vi "DDC Stage 02 - Single channel.vi"(0 "input cluster":T1={"acq.reset"=FALSE, "ddc.out.rate"=[0.0, 0.0, 0.0, 0.0, 0.0, 0.0, 0.0, 0.0, 0.0, 0.0, 0.0, 0.0, 0.0, 0.0, 0.0, 0.0], "ddc.delay"=[0.0, 0.0, 0.0, 0.0, 0.0, 0.0, 0.0, 0.0, 0.0, 0.0, 0.0, 0.0, 0.0, 0.0, 0.0, 0.0], "Channel#"=0} {"ddc.out.rate" format="%.48g"; "ddc.delay" format="%.16g"}, 7 "FIFO In":refnum<k21>="FIFO-000", 11 "Ch#":u8) -> (3 "dsp.overflow":bool, 4 "U32 out":u32, 10 "output valid":bool, 14 "dbg,output1":T2)   [LabVIEW 2015, in "DDC_7976R_v1.lvlib"]
uses:
  DDC_7976R_v1.lvlib
  Typedef - internal -03.ctl
  Typedef - internal -04.ctl
  <instrlib>/_niInstr/DSP/v1/FPGA/Public/Sub VIs/HB Decimator/Halfband Decimator - IQ - 16 spc - 2x oc.vi
  <instrlib>/_niInstr/DSP/v1/FPGA/Public/Sub VIs/HB Decimator/Halfband Decimator - IQ - 8 spc - 2x oc.vi
  <instrlib>/_niInstr/DSP/v1/FPGA/Public/Sub VIs/HB Decimator/Halfband Decimator - IQ - 4 spc - 2x oc.vi
  <instrlib>/_niInstr/DSP/v1/FPGA/Public/Sub VIs/HB Decimator/Halfband Decimator - IQ - 2 spc - 2x oc.vi
  <instrlib>/_niInstr/DSP/v1/FPGA/Public/Sub VIs/Fractional Decimator/Fractional Decimator - 1 spc - 2x oc.vi
  <instrlib>/_niInstr/DSP/v1/Xnodes/Public/Decimator/niInstr DSP v1 Decimator FPGA.xnode
  <instrlib>/_niInstr/DSP/v1/Shared/Public/IQ Data.ctl
  <instrlib>/_niInstr/DSP/v1/FPGA/niInstr DSP v1 FPGA.lvlib
  <instrlib>/_niInstr/DSP/v1/Shared/niInstr DSP v1 Shared.lvlib
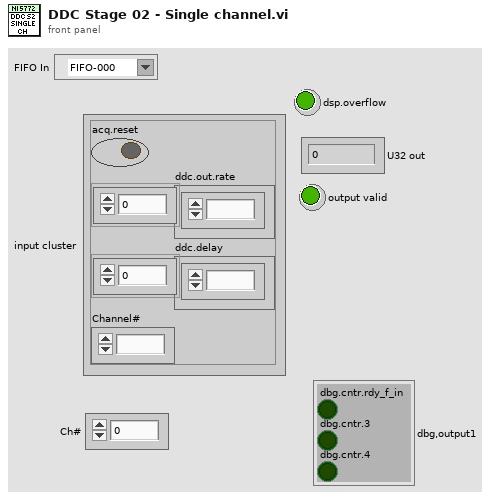
[diagram p1: front panel]
types:
  T1 = typedef "DDC_7976R_v1.lvlib/Typedef - internal -04.ctl" = cluster{"acq.reset":bool, "ddc.out.rate":fxp<+,48,1>[], "ddc.delay":fxp<+/-,16,0>[], "Channel#":u8}
  T2 = typedef "DDC_7976R_v1.lvlib/Typedef - internal -03.ctl" = cluster{"dbg.cntr.4":bool, "dbg.cntr.3":bool, "dbg.cntr.rdy_f_in":bool}
  T3 = cluster{"I":fxp<+/-,18,1>, "Q":fxp<+/-,18,1>, "overflow":bool}[]
  T4 = typedef "niInstr DSP v1 Shared.lvlib/IQ Data.ctl" = cluster{"I":fxp<+/-,18,1>, "Q":fxp<+/-,18,1>, "overflow":bool}
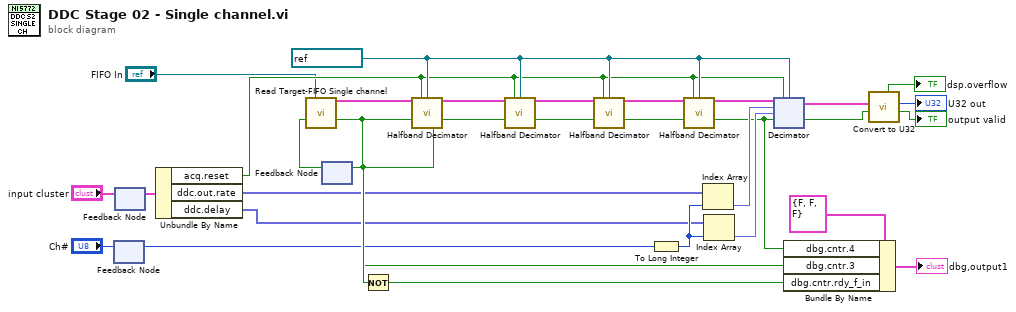
[diagram p0: block diagram]
diagram:
  w14 = refnum<k21> "204MHz" ("Refnum in")
  n1 = feedback #1() -> (w2:u8)  [unwired: 1 in]
  n2 = feedback-in #1("Ch#") -> ()
  n3 = feedback-in #2("input cluster") -> ()
  n4 = feedback #2() -> (w9:T1)  [unwired: 1 in]
  n5 = Unbundle By Name(w9) -> ("acq.reset"=w11:bool, "ddc.out.rate"=w12:fxp<+,48,1>[], "ddc.delay"=w13:fxp<+/-,16,0>[])
  n6 = feedback #3() -> (w32:bool)  [unwired: 1 in]
  n7 = call "Read Target-FIFO Single channel.vi"("FIFO In"="FIFO In", "ready for input"=w32) -> ("16xIQData"=w30:T3, "Output Valid"=w17:bool)  [unwired: 12 in]
  n8 = call-poly <instrlib>:"Halfband Decimator.vi"("data in"=w30, "reset"=w11, "clock x 2"=w14, "input valid"=w17) -> ("data out"=w21:T4[], "output valid"=w22:bool, "ready for input"=w31:bool)  [unwired: 9 in]
  n9 = feedback-in #3(w31) -> ()
  n10 = Not(x=w31) -> (.not. x?=w18:bool)
  n11 = call-poly <instrlib>:"Halfband Decimator.vi"("data in"=w21, "reset"=w11, "clock x 2"=w14, "input valid"=w22) -> ("data out"=w23:T4[], "output valid"=w24:bool)  [unwired: 9 in, 1 out]
  n12 = call-poly <instrlib>:"Halfband Decimator.vi"("data in"=w23, "reset"=w11, "clock x 2"=w14, "input valid"=w24) -> ("data out"=w25:T4[], "output valid"=w27:bool)  [unwired: 9 in, 1 out]
  n13 = To Long Integer(number=w2) -> (32bit integer=w20:i32)
  n14 = call-poly <instrlib>:"Halfband Decimator.vi"("data in"=w25, "reset"=w11, "clock x 2"=w14, "input valid"=w27) -> ("data out"=w26:T4, "output valid"=w16:bool)  [unwired: 9 in, 1 out]
  n15 = Index Array(array=w12, index=w20) -> (element=w29:fxp<+,48,1>)
  n16 = Index Array(array=w13, index=w20) -> (element=w28:fxp<+/-,16,0>)
  n17 = xnode "Decimator"("data in"=w26, "reset"=w11, "input valid"=w16, "output sample rate"=w29, "delay"=w28, "clock x2"=w14) -> ("data out"=w7:T4, "output valid"=w6:bool)  [unwired: 1 out]
  n18 = Bundle By Name(cluster=T2 {"dbg.cntr.4"=FALSE, "dbg.cntr.3"=FALSE, "dbg.cntr.rdy_f_in"=FALSE} ("output cluster"), "dbg.cntr.4"=w16, "dbg.cntr.3"=w17, "dbg.cntr.rdy_f_in"=w18) -> (→"dbg,output1":T2)
  n19 = call "Convert to U32.vi"("input valid"=w6, "IQData in"=w7) -> ("output valid"=→"output valid":bool, "U32 out"=→"U32 out":u32, "overflow"=→"dsp.overflow":bool)  [unwired: 7 in]
